vi "Utility Write To Register - Integers.vi"(0 "VISA resource name":refnum<visa-resource-name>, 1 "Unit Address (1)":u8=1, 5 "Register Address (0)":u16, 9 "Data (0)":i16, 11 "error in (no error)":errorcluster) -> (4 "VISA resource name out":refnum<visa-resource-name>, 15 "error out":errorcluster {"code" format="%.0x"})   [LabVIEW 2010, in "Eurotherm 32xx Series.lvlib"]
doc: "This VI writes the value to the specified register of specified unit."
uses:
  <instrlib>/Eurotherm 32xx Series/Eurotherm 32xx Series.lvlib
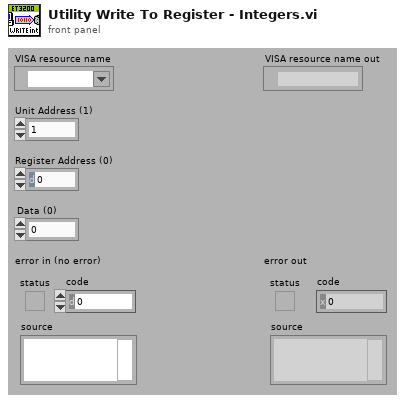
[diagram p1: front panel]
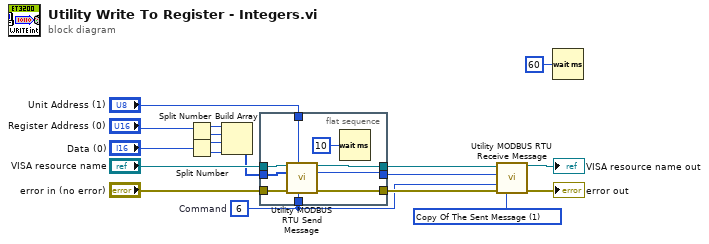
[diagram p0: block diagram]
diagram:
  w1 = u16 1 items=["By The Number Of Bytes", "Copy Of The Sent Message"] ("Receive Message Type (0: By The Number Of Bytes)")
  w12 = u8 6  # Command
  n1 = Split Number(x="Register Address (0)") -> (hi(x)=w10:u8, lo(x)=w9:u8)
  n2 = Split Number(x="Data (0)") -> (hi(x)=w8:u8, lo(x)=w7:u8)
  n3 = Build Array(w10, w9, w8, w7) -> (w11:u8[])
  n4 = flat-sequence {
    tunnel: "VISA resource name" -> [w27]
    tunnel: "error in (no error)" -> [w26]
    tunnel: [w25] -> w14
    tunnel: [w24] -> w13
    tunnel: w12 -> [w23]
    tunnel: w11 -> [w22]
    tunnel: [w21] -> w6
    tunnel: "Unit Address (1)" -> [w20]
    frame #0 {
      n5 = call <instrlib>:"Utility MODBUS RTU Send Message.vi"("VISA resource name"=w27, "Unit Address (1)"=w20, "Message (empty array)"=w22, "error in (no error)"=w26, "Command (0)"=w23) -> ("VISA resource name out"=w24:refnum<visa-resource-name>, "Length Of Sent MSG"=w21:u8, "error out"=w25:errorcluster)  [unwired: 8 in]
      n6 = Wait (ms)(milliseconds to wait=u32 10) -> ()  [unwired: 1 out]
    }
  }
  n7 = call <instrlib>:"Utility MODBUS RTU Receive Message.vi"("VISA resource name"=w13, "Length Of Sent MSG (0)"=w6, "Sent Command (0)"=w12, "error in (no error)"=w14, "Receive Message Type (0: By The Number Of Bytes)"=w1) -> ("VISA resource name out"=→"VISA resource name out":refnum<visa-resource-name>, "error out"=→"error out":errorcluster)  [unwired: 8 in, 1 out]
  n8 = Wait (ms)(milliseconds to wait=u32 60) -> ()  [unwired: 1 out]
